vi "ParseArguments.vi"(8 "error in (no error)":errorcluster, 10 "Inputs":string[](array[string]), 11 "RunVI in":refnum<class "RunVI.lvclass">) -> (0 "error out":errorcluster, 3 "RunVI out":refnum<class "RunVI.lvclass">)   [LabVIEW 2014, in "RunVI.lvclass"]
uses:
  RunVI.lvclass
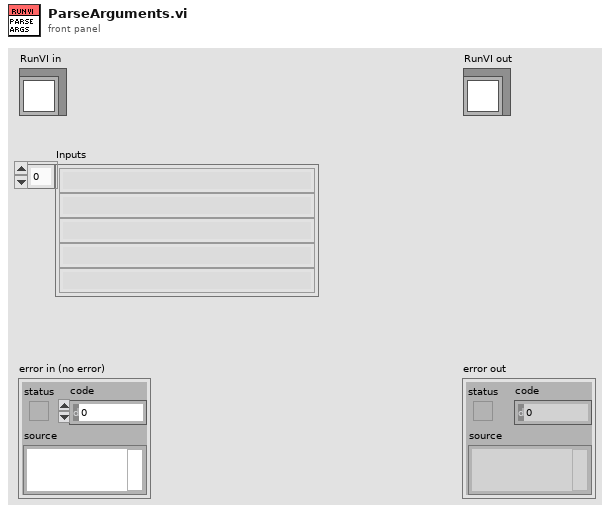
[diagram p1: front panel]
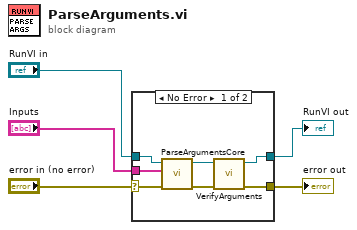
[diagram p0: block diagram]
diagram:
  n1 = case shown="No Error" "error in (no error)" {
    selector: "error in (no error)" -> [w10 w14]
    tunnel: [w8 w14] -> w4
    tunnel: [w6 w13] -> w1
    tunnel: "RunVI in" -> [w12 w13]
    tunnel: "Inputs" -> [w11 _]
    frame No Error {
      n2 = call "ParseArgumentsCore.vi"("error in (no error)"=w10, "Inputs"=w11, "RunVI in"=w12) -> ("error out"=w9:errorcluster, "RunVI out"=w7:refnum<class "RunVI.lvclass">)  [unwired: 7 in]
      n3 = call "VerifyArguments.vi"("error in (no error)"=w9, "RunVI in"=w7) -> ("error out"=w8:errorcluster, "RunVI out"=w6:refnum<class "RunVI.lvclass">)  [unwired: 8 in]
    }
    frame Error {
    }
  }
  "error out" <- w4
  "RunVI out" <- w1
